vi "TR_DRAW_Track_overlays_(offline).vi"(0 "Image size":cluster{"x":i32, "y":i32}={"x"=480, "y"=480}, 1 "Overlays cluster in":T1, 5 "Full track array":T2, 11 "Error In":errorcluster) -> (4 "Overlays cluster out":T1, 15 "Error Out":errorcluster)   [LabVIEW 2018, in "Tracks Repair.lvlib"]
uses:
  Tracks Repair.lvlib
  SubVi's/Controls/CTL_Full_Track_Array.ctl
  SubVi's/Controls/CTL_Overlays_cluster.ctl
  Tracker.lvlib
panel:
  in  "Lower bound":cluster{"x":i32, "y":i32}
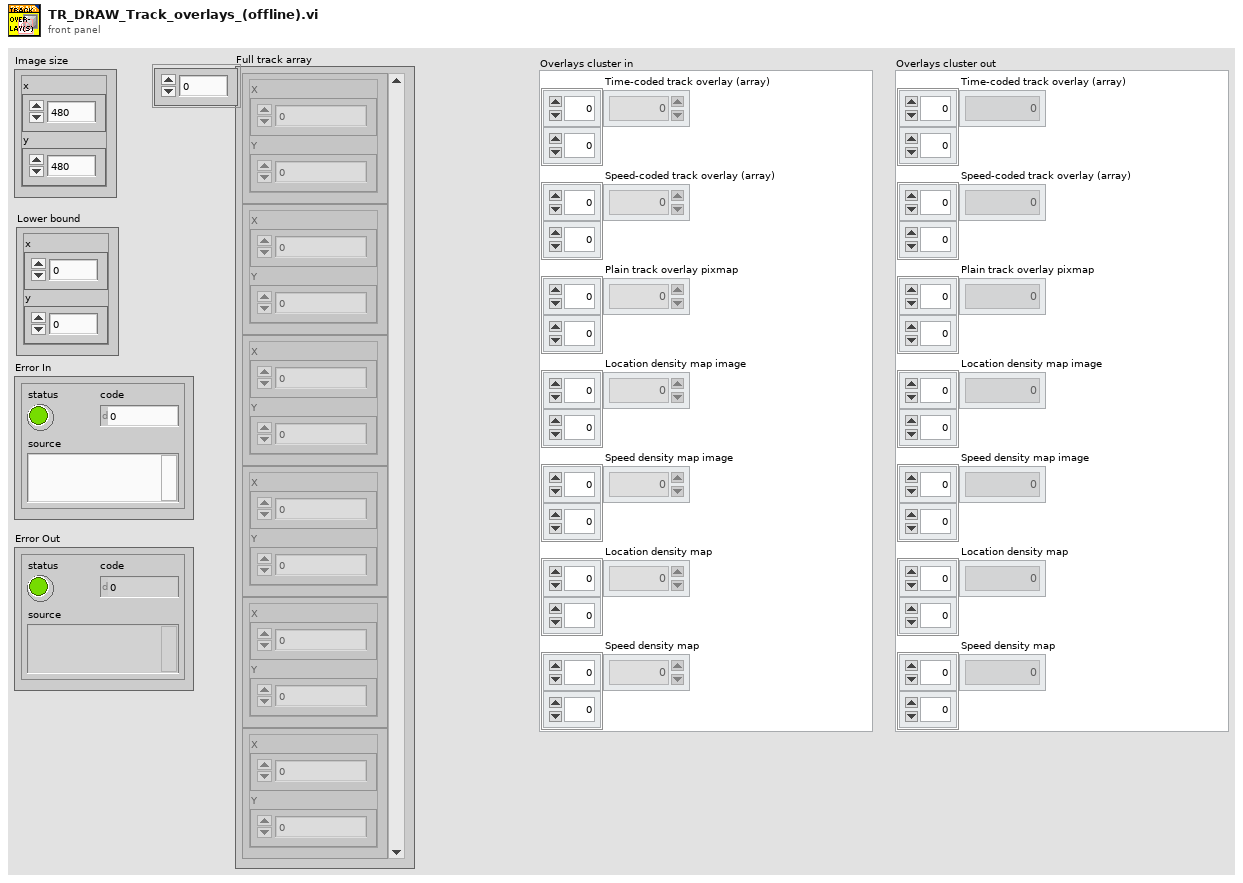
[diagram p1: front panel]
types:
  T1 = typedef "Tracker.lvlib/CTL_Overlays_cluster.ctl" = cluster{"Time-coded track overlay (array)":u32[][], "Speed-coded track overlay (array)":u32[][], "Plain track overlay pixmap":u32[][], "Location density map image":u32[][], "Speed density map image":u32[][], "Location density map":dbl[][], "Speed density map":dbl[][]}
  T2 = typedef "Tracker.lvlib/CTL_Full_Track_Array.ctl" = cluster{"X":dbl, "Y":dbl}[]
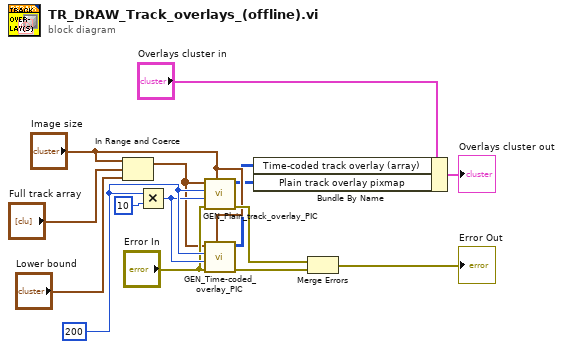
[diagram p0: block diagram]
diagram:
  w12 = 200 ("Multiline grouping")
  n1 = In Range and Coerce(upper limit="Image size", x="Full track array", lower limit="Lower bound") -> (coerced(x)=w8:cluster{"X":dbl, "Y":dbl}[])  [unwired: 1 out]
  n2 = Multiply(x=w12, y=10) -> (x*y=w11:i32)
  n3 = call "GEN_Plain_track_overlay_PIC.vi"("Image size"="Image size", "Error In"="Error In", "Samples full merge, every N"=w11, "Multiline grouping, samples"=w12, "Full track array"=w8) -> ("Error Out"=w9:errorcluster, "Plain track overlay pixmap"=w1:u32[][])  [unwired: 5 in]
  n4 = call "GEN_Time-coded_overlay_PIC.vi"("Image size"="Image size", "Error In"="Error In", "Samples full merge, every N"=w11, "Multiline grouping, samples"=w12, "Full track array"=w8) -> ("Error Out"=w13:errorcluster, "Time-coded overlay pixmap"=w2:u32[][])  [unwired: 5 in]
  n5 = Bundle By Name(cluster="Overlays cluster in", "Time-coded track overlay (array)"=w2, "Plain track overlay pixmap"=w1) -> (→"Overlays cluster out":T1)
  n6 = Merge Errors(w9, w13) -> (→"Error Out":errorcluster)
